vi "Read Error Cluster Attribute.vi"(10 "attribute name":string, 11 "error":errorcluster) -> (1 "found?":bool, 2 "value string":string, 3 "JSON object string":string)   [LabVIEW 2020, in "Multi Error Cluster.lvlib"]
doc: "Returns the value of an attribute stored in an error cluster. If the attribute is not found, this VI returns an empty string."
uses:
  <vilib>/MultiError/TokenizeJSON/Multi Error Cluster.lvlib
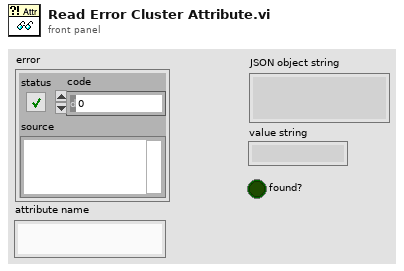
[diagram p1: front panel]
types:
  T1 = typedef "Multi Error Cluster.lvlib/JSON Token Values.ctl" = enum32{"array begin", "array end", "object begin", "object end", "value", "invalid", "name"}
  T2 = typedef "Multi Error Cluster.lvlib/JSON Token Descriptor.ctl" = cluster{"match string":string, "raw token type":T3, "byte offset ":i32}
  T3 = typedef "Multi Error Cluster.lvlib/JSON Raw Token Values.ctl" = enum32{"{", "}", "[", "]", ",", ":", "\"", "number", "string", "true", "false", "null", "invalid"}
  T4 = typedef "Multi Error Cluster.lvlib/JSON Object Descriptor.ctl" = cluster{"begin info":T2, "end info":T2, "begin Index":i32, "end Index":i32}
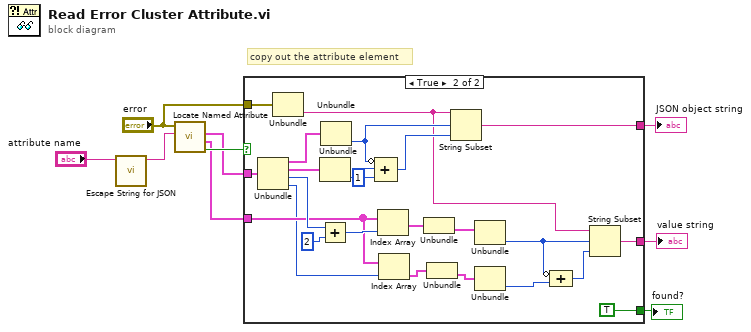
[diagram p0: block diagram]
diagram:
  # "copy out the attribute element"
  n1 = call <vilib>:"Escape String for JSON.vi"("string"="attribute name") -> ("quoted string"=w1:string)  [unwired: 10 in]
  n2 = call <vilib>:"Locate Named Attribute.vi"("attribute name"=w1, "error"="error") -> ("found"=w6:bool, "attribute tokens"=w4:cluster{"token type":T1, T2}[], "JSON Object Descriptor"=w5:T4)  [unwired: 5 in, 2 out]
  n3 = case shown="True" w6 {
    tunnel: [_ w25] -> w9
    tunnel: [_ TRUE] -> w8
    tunnel: w5 -> [_ w32]
    tunnel: "error" -> [_ w29]
    tunnel: w4 -> [_ w18]
    tunnel: [_ w11] -> w3
    frame False {
    }
    frame True {
      n4 = Unbundle(w32) -> ("begin info"=w31:T2, "end info"=w30:T2, "begin Index"=w21:i32, "end Index"=w10:i32)
      n5 = Unbundle(w29) -> ("source"=w15:string)  [unwired: 2 out]
      n6 = Unbundle(w30) -> ("byte offset"=w28:i32)  [unwired: 2 out]
      n7 = Add(x=w21, y=2 ("value")) -> (x+y=w23:i32)
      n8 = Unbundle(w31) -> ("byte offset"=w27:i32)  [unwired: 2 out]
      n9 = Compound Arithmetic op=ADD(invert w27, w28, 1 ("value")) -> (w26:i32)
      n10 = Index Array(array=w18, index=w23) -> (element=w22:cluster{"token type":T1, T2})
      n11 = Index Array(array=w18, index=w10) -> (element=w19:cluster{"token type":T1, T2})
      n12 = Unbundle(w22) -> (w17:T2)  [unwired: 1 out]
      n13 = Unbundle(w19) -> (w16:T2)  [unwired: 1 out]
      n14 = String Subset(string=w15, offset (0)=w27, length (rest)=w26) -> (substring=w25:string)
      n15 = Unbundle(w17) -> ("byte offset"=w14:i32)  [unwired: 2 out]
      n16 = Unbundle(w16) -> ("byte offset"=w13:i32)  [unwired: 2 out]
      n17 = Compound Arithmetic op=ADD(invert w14, w13) -> (w12:i32)
      n18 = String Subset(string=w15, offset (0)=w14, length (rest)=w12) -> (substring=w11:string)
    }
  }
  "JSON object string" <- w9
  "found?" <- w8
  "value string" <- w3
